vi "fileweek05.vi"() -> ()   [LabVIEW 2021]
uses:
  <vilib>/Utility/file.llb/Write Delimited Spreadsheet (DBL).vi
panel:
  in  "Path to save file":path
  out "Waveform Graph":dbl[][](graph)
  out "Data":dbl[](array[numeric])
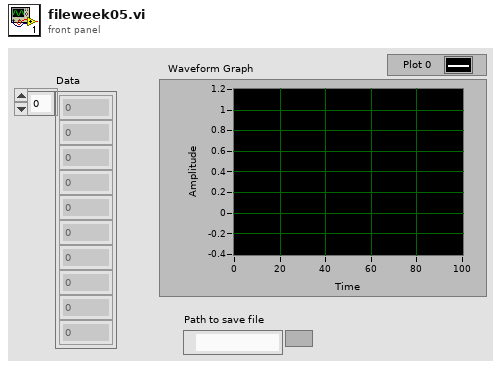
[diagram p1: front panel]
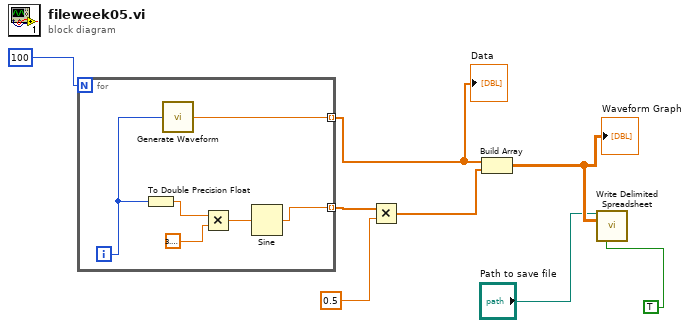
[diagram p0: block diagram]
diagram:
  n1 = for {
    N: 100 -> [_]
    tunnel: [w10] -> w6 mode=indexing
    tunnel: [w9] -> w7 mode=indexing
    i -> [w14]
    n2 = To Double Precision Float(number=w14) -> (double precision float=w12:dbl)
    n3 = call "Generate Waveform.vi"("Index"=w14) -> ("Waveform Point"=w9:dbl)
    n4 = Multiply(x=w12, y=3.141592653589793) -> (x*y=w11:dbl)
    n5 = Sine(x=w11) -> (sin(x)=w10:dbl)
  }
  "Data" <- w7
  n6 = Multiply(x=w6, y=0.5) -> (x*y=w4:dbl[])
  n7 = Build Array(w7, w4) -> (w3:dbl[][])
  "Waveform Graph" <- w3
  n8 = call-poly <vilib>:"Write Delimited Spreadsheet.vi"("file path (dialog if empty)"="Path to save file", "2D data"=w3, "transpose? (no:F)"=TRUE) -> ()  [unwired: 11 in, 2 out]
